vi "write_out_bit.vi"() -> ()   [LabVIEW 2012]
uses:
  Usb_Daq_V52_Dll.dll
panel:
  in  "端口号":i8 min=0 max=15 step=1
  in  "stop":bool
  in  "OUT":bool
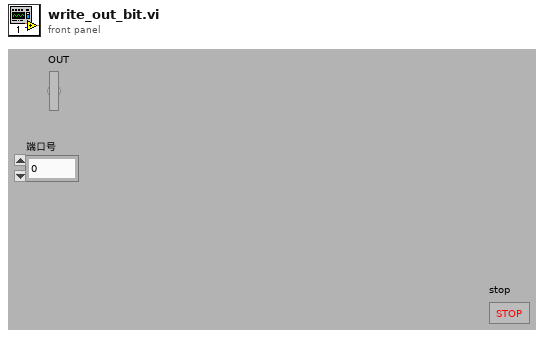
[diagram p1: front panel]
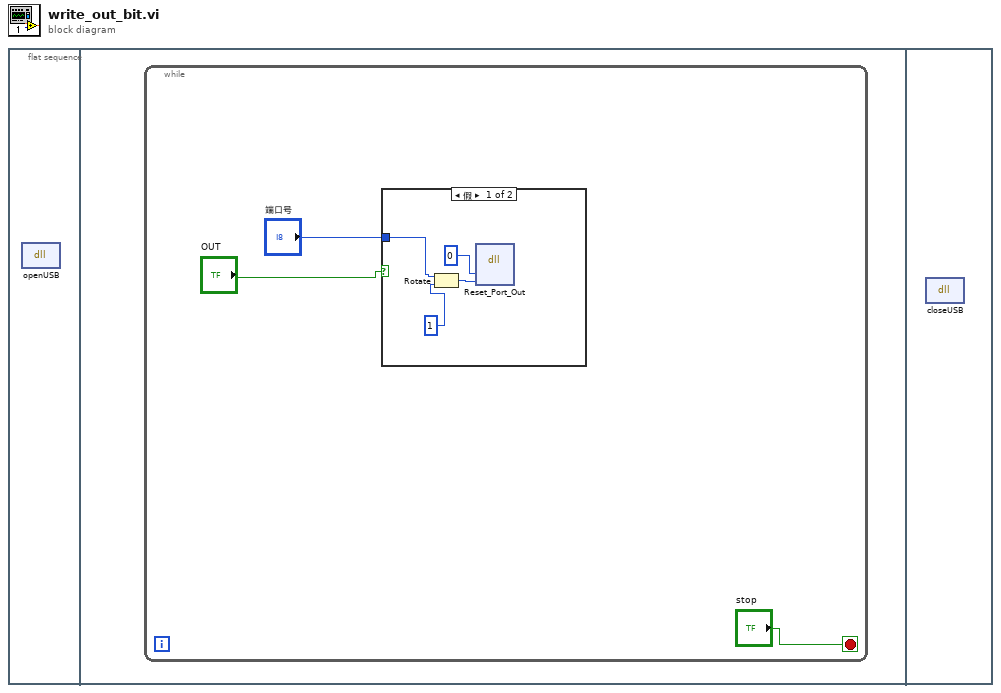
[diagram p0: block diagram]
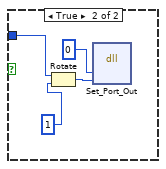
[diagram p2: hidden frame]
diagram:
  n1 = flat-sequence {
    frame #0 {
      n2 = dll-call lib="PTH1labs Ebackup数据采集卡uSB!USB数据采集卡资料HKUSB6203例程labviewUsb_Daq_V52_Dll.dll" fn="openUSB"() -> ()  [unwired: 3 in, 3 out]
    }
    frame #1 {
      n3 = while {
        stop <- "stop" stop-if-true
        n4 = case shown="假" "OUT" {
          tunnel: "端口号" -> [w5 w9]
          frame False {
            n5 = Rotate(1:1, 2:w5) -> (0:w6:i32)
            n6 = dll-call lib="PTH1labs Ebackup数据采集卡uSB!USB数据采集卡资料HKUSB6203例程labviewUsb_Daq_V52_Dll.dll" fn="Reset_Port_Out"("dev"=0, "参数1"=w6) -> ()  [unwired: 3 in, 5 out]
          }
          frame True {
            n7 = Rotate(1:1, 2:w9) -> (0:w10:i32)
            n8 = dll-call lib="PTH1labs Ebackup数据采集卡uSB!USB数据采集卡资料HKUSB6203例程labviewUsb_Daq_V52_Dll.dll" fn="Set_Port_Out"("dev"=0, "参数1"=w10) -> ()  [unwired: 3 in, 5 out]
          }
        }
      }
    }
    frame #2 {
      n9 = dll-call lib="PTH1labs Ebackup数据采集卡uSB!USB数据采集卡资料HKUSB6203例程labviewUsb_Daq_V52_Dll.dll" fn="closeUSB"() -> ()  [unwired: 3 in, 3 out]
    }
  }
